vi "Port Speed to String.vi"(8 "error in":errorcluster, 11 "port":T1 format="%.0x") -> (0 "error out":errorcluster, 1 "speed string":string, 2 "mode string":string, 3 "port out":T1 format="%.0x")   [LabVIEW 2020, in "Ballard ARINC 429 Hardware Configuration.lvlib"]
uses:
  Ballard ARINC 429 Hardware Configuration.lvlib
  Scripting/Ballard/Ballard ARINC 429 Scripting.lvlib
  Shared/Transfer Speed.ctl
  <vilib>/NI VeriStand/Custom Device API/Custom Device Item Ref.ctl
  <vilib>/NI VeriStand/Custom Device API/Custom Device API.lvlib
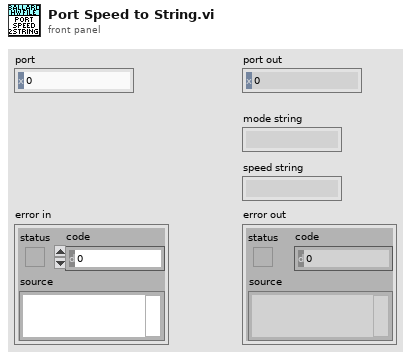
[diagram p1: front panel]
types:
  T1 = typedef "Custom Device API.lvlib/Custom Device Item Ref.ctl" = u64
  T2 = typedef "Transfer Speed.ctl" = enum16{"LO (12.5 kb/s)", "HI (100 kb/s)"}
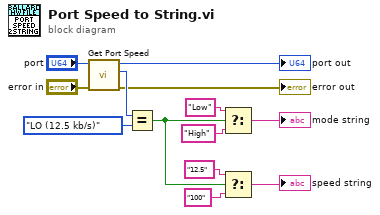
[diagram p0: block diagram]
diagram:
  n1 = call "Get Port Speed.vi"("error in"="error in", "port ref"="port") -> ("error out"=→"error out":errorcluster, "speed"=w9:T2, "port ref out"=→"port out":T1)  [unwired: 7 in]
  n2 = Equal?(x=w9, y=Transfer_Speed."LO (12.5 kb/s)") -> (x = y?=w4:bool)
  n3 = Select(t="Low", s=w4, f="High") -> (s? t:f=→"mode string":string)
  n4 = Select(t="12.5", s=w4, f="100") -> (s? t:f=→"speed string":string)
